vi "initialize arrays.vi"(10 "Game Parameters":T3={"Upper Limit (m)"=100.0, "Lower Limit (m)"=0.0, "Obstacle time"=20.0, "Obstacle length"=10.0, "fuel decrement"=0.5, "Fuel time"=100.0, "fuel amount"=50.0, "Fuel range"=10, "Death range"=5, "Terrain slope"=35.0, "Speed (km/hr)"=150.0, "Time step (ms)"=30, "Gravity"=-9.81, "Date"="11/03/2016", "High scores path"=path "C:/Users/lz2/Code/LabVIEW/Helicopter/hi scores.txt", "Difficulty"=enum."Normal", "Headstart"=30}, 11 "Arrays and Heights":T1={"Score Array"=[], "Lowest high score"=0.0, "Score"=0.0, "Ceiling"=0.0, "Floor"=0.0, "Ceiling Array"=[], "Floor array"=[], "Helicopter height"=0.0, "Helicopter array"=[], "Fuel"=300.0, "Fuel array"=[], "fuel counter"=0, "obstacle counter"=0, "Obstacle array"=[], "helicopter v_0"=0.0, "helicopter a_0"=0.0, "Obstacle height"=300.0}) -> (3 "Arrays and values":T1={"Score Array"=[], "Lowest high score"=0.0, "Score"=0.0, "Ceiling"=0.0, "Floor"=0.0, "Ceiling Array"=[], "Floor array"=[], "Helicopter height"=0.0, "Helicopter array"=[], "Fuel"=300.0, "Fuel array"=[], "fuel counter"=0, "obstacle counter"=0, "Obstacle array"=[], "helicopter v_0"=0.0, "helicopter a_0"=0.0, "Obstacle height"=300.0})   [LabVIEW 2017]
uses:
  controls/arrays and heights.ctl
  controls/scores.ctl
  controls/game parameters.ctl
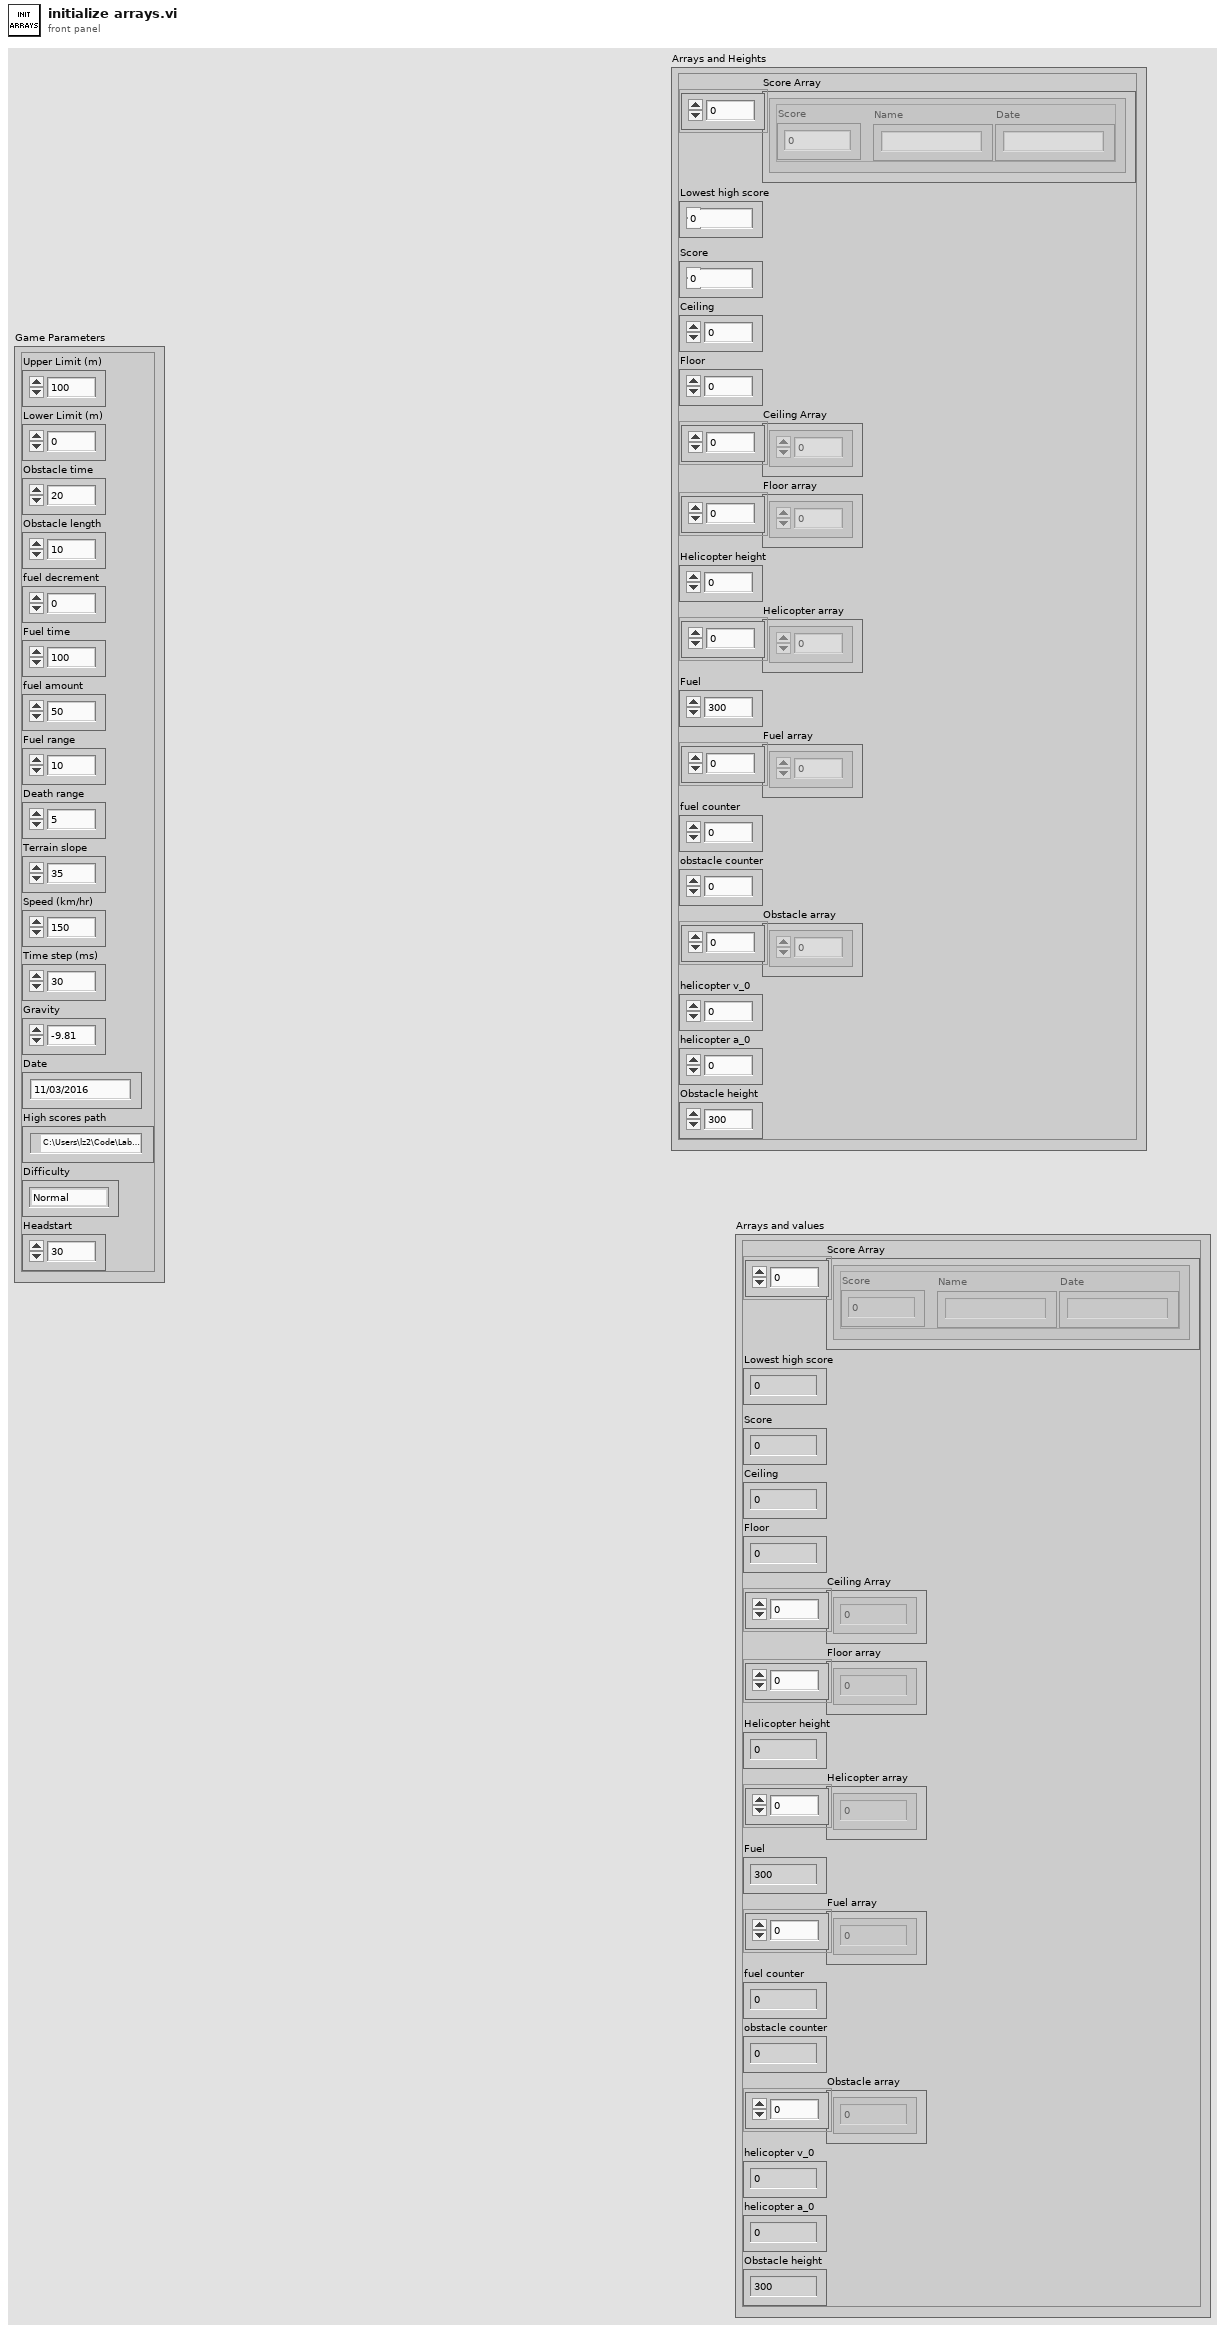
[diagram p1: front panel]
types:
  T1 = typedef "arrays and heights.ctl" = cluster{"Score Array":T2[], "Lowest high score":dbl, "Score":dbl, "Ceiling":dbl, "Floor":dbl, "Ceiling Array":dbl[], "Floor array":dbl[], "Helicopter height":dbl, "Helicopter array":dbl[], "Fuel":dbl, "Fuel array":dbl[], "fuel counter":i32, "obstacle counter":i32, "Obstacle array":dbl[], "helicopter v_0":dbl, "helicopter a_0":dbl, "Obstacle height":dbl}
  T2 = typedef "scores.ctl" = cluster{"Score":dbl, "Name":string, "Date":string}
  T3 = typedef "game parameters.ctl" = cluster{"Upper Limit (m)":dbl, "Lower Limit (m)":dbl, "Obstacle time":dbl, "Obstacle length":dbl, "fuel decrement":dbl, "Fuel time":dbl, "fuel amount":dbl, "Fuel range":i32, "Death range":i32, "Terrain slope":dbl, "Speed (km/hr)":dbl, "Time step (ms)":u32, "Gravity":dbl, "Date":string, "High scores path":path, "Difficulty":enum16{"Easy", "Normal", "Hard"}, "Headstart":u32}
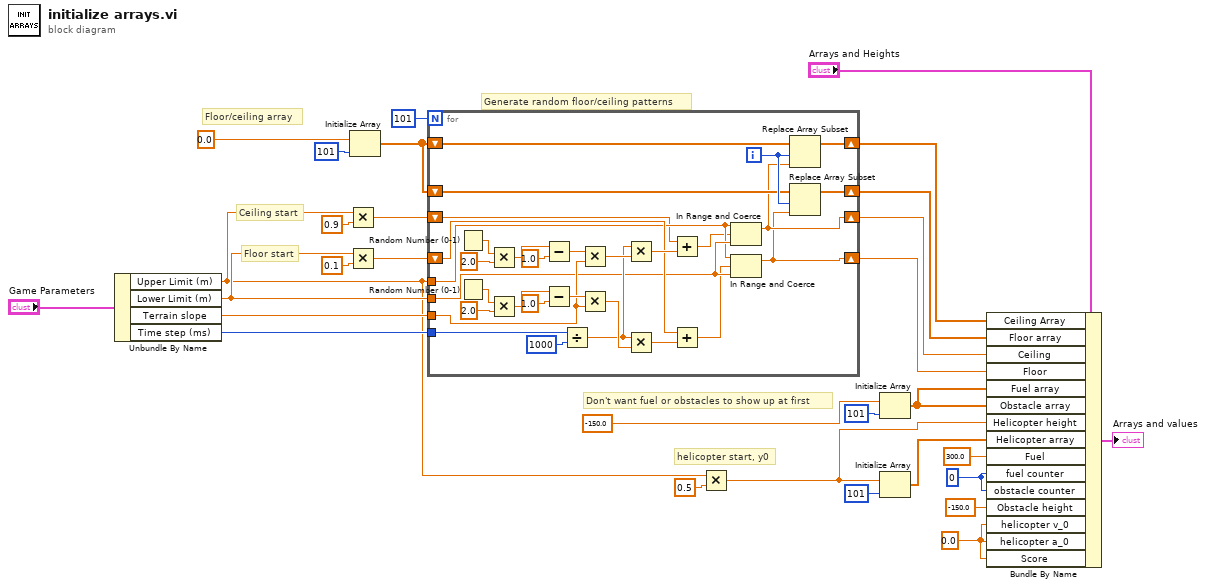
[diagram p0: block diagram]
diagram:
  w1 = 0.0 ("helicopter v_0")
  w3 = 0 ("fuel counter")
  # "helicopter start, y0"
  # "Don't want fuel or obstacles to show up at first"
  # "Floor start"
  # "Ceiling start"
  # "Generate random floor/ceiling patterns"
  # "Floor/ceiling array"
  n1 = Unbundle By Name("Game Parameters") -> ("Upper Limit (m)"=w8:dbl, "Lower Limit (m)"=w15:dbl, "Terrain slope"=w29:dbl, "Time step (ms)"=w28:u32)
  n2 = Multiply(x=w8, y=0.9) -> (x*y=w18:dbl)
  n3 = Multiply(x=w15, y=0.1) -> (x*y=w19:dbl)
  n4 = Initialize Array(0.0 ("element"), 101 ("dimension size")) -> (w20:dbl[])
  n5 = for {
    N: 101 -> [_]
    tunnel: w29 -> [w47]
    tunnel: w28 -> [w45]
    shift-right: [w32] -> w27
    shift-left: w18 -> [w33]
    shift-right: [w31] -> w26
    shift-left: w19 -> [w38]
    shift-right: [w40] -> w17
    shift-left: w20 -> [w41]
    shift-right: [w39] -> w16
    shift-left: w20 -> [w42]
    tunnel: w8 -> [w36]
    tunnel: w15 -> [w37]
    i -> [w43]
    n6 = Random Number (0-1)() -> (number: 0 to 1=w57:dbl)
    n7 = Random Number (0-1)() -> (number: 0 to 1=w51:dbl)
    n8 = Multiply(x=w57, y=2.0) -> (x*y=w59:dbl)
    n9 = Multiply(x=w51, y=2.0) -> (x*y=w49:dbl)
    n10 = Subtract(x=w59, y=1.0) -> (x-y=w56:dbl)
    n11 = Subtract(x=w49, y=1.0) -> (x-y=w52:dbl)
    n12 = Divide(x=w45, y=u32 1000) -> (x/y=w44:dbl)
    n13 = Multiply(x=w56, y=w47) -> (x*y=w55:dbl)
    n14 = Multiply(x=w52, y=w47) -> (x*y=w53:dbl)
    n15 = Multiply(x=w44, y=w55) -> (x*y=w61:dbl)
    n16 = Multiply(x=w44, y=w53) -> (x*y=w54:dbl)
    n17 = Add(x=w33, y=w61) -> (x+y=w35:dbl)
    n18 = Add(x=w38, y=w54) -> (x+y=w34:dbl)
    n19 = In Range and Coerce(upper limit=w36, x=w35, lower limit=w37) -> (coerced(x)=w32:dbl)  [unwired: 1 out]
    n20 = In Range and Coerce(upper limit=w36, x=w34, lower limit=w37) -> (coerced(x)=w31:dbl)  [unwired: 1 out]
    n21 = Replace Array Subset(array=w41, new element=w32, index=w43) -> (w40:dbl[])
    n22 = Replace Array Subset(array=w42, new element=w31, index=w43) -> (w39:dbl[])
  }
  n23 = Multiply(x=w8, y=0.5 ("Helicopter start (m)")) -> (x*y=w7:dbl)
  n24 = Initialize Array(-150.0 ("element"), 101 ("dimension size")) -> (w10:dbl[])
  n25 = Initialize Array(w7, 101 ("dimension size")) -> (w5:dbl[])
  n26 = Bundle By Name(cluster="Arrays and Heights", "Ceiling Array"=w17, "Floor array"=w16, "Ceiling"=w27, "Floor"=w26, "Fuel array"=w10, "Obstacle array"=w10, "Helicopter height"=w7, "Helicopter array"=w5, "Fuel"=300.0 ("Fuel amount"), "fuel counter"=w3, "obstacle counter"=w3, "Obstacle height"=-150.0, "helicopter v_0"=w1, "helicopter a_0"=w1, "Score"=w1) -> (→"Arrays and values":T1)
